vi "AI Driver Initialize.vi"(8 "error in (no error)":errorcluster, 11 "Channel Refs":T3[](array[typedef]) format="%.0x") -> (0 "error out":errorcluster, 3 "Tasks":T1[](array[typedef]))   [LabVIEW 2013]
uses:
  <vilib>/K2Labs/HiLab API/Custom Device API/Controls/Custom Device Item Reference.ctl
  Controls/AI Device Settings.ctl
  Controls/AI Scale.ctl
  <vilib>/K2Labs/HiLab API/Custom Device API/Configuration/Item Properties/Get Item Property/Get Item Property.xnode
  <vilib>/K2Labs/HiLab API/Custom Device API/Custom Device API Library.lvlib
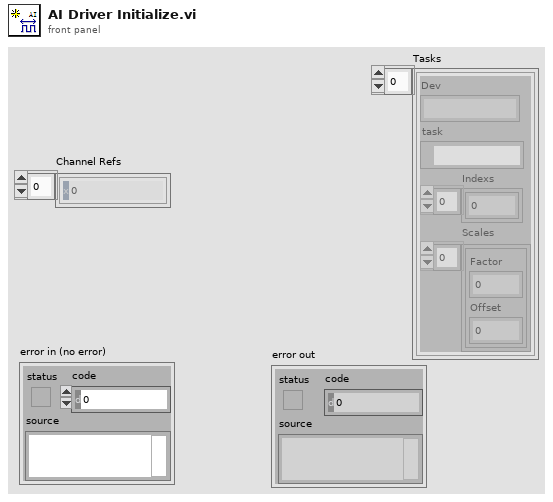
[diagram p1: front panel]
types:
  T1 = typedef "AI Device Settings.ctl" = cluster{"Dev":string, "task":refnum<k21>, "Indexs":i32[], "Scales":T2[]}
  T2 = typedef "AI Scale.ctl" = cluster{"Factor":dbl, "Offset":dbl}
  T3 = typedef "Custom Device API Library.lvlib/Custom Device Item Reference.ctl" = u64
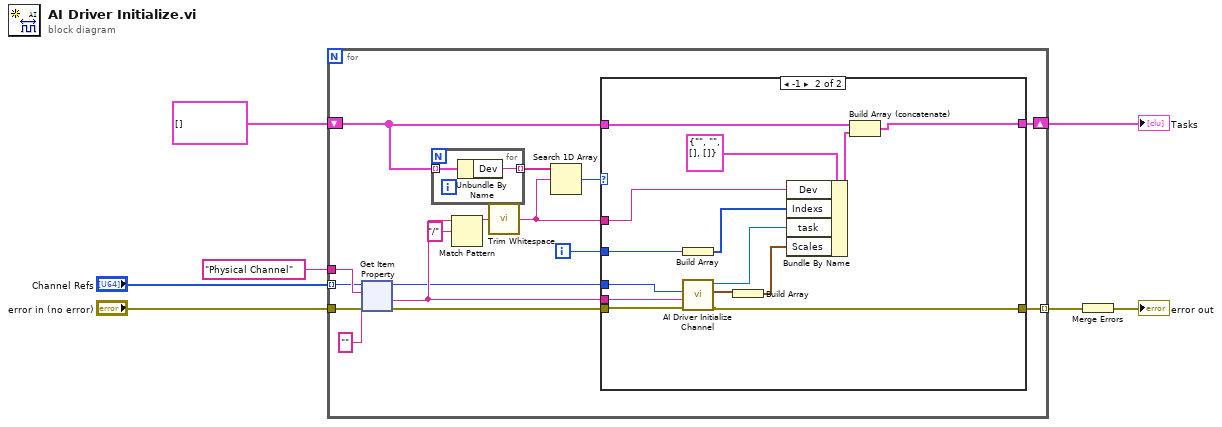
[diagram p0: block diagram]
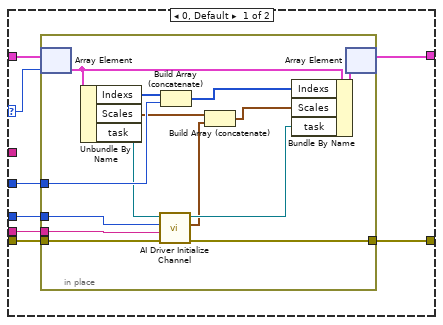
[diagram p2: hidden frame]
diagram:
  n1 = for {
    tunnel: "Physical Channel" ("Property Name") -> [w23]
    tunnel: "Channel Refs" -> [w22] mode=indexing
    shift-right: [w16] -> w1
    shift-left: T1[] [] -> [w17]
    tunnel: [w11] -> w3 mode=indexing
    tunnel: "error in (no error)" -> [w10]
    i -> [w12]
    n2 = xnode "Get Item Property"("Item Ref in"=w22, "Property Name"=w23, "Default Value"="", "error in (no error)"=w10) -> ("Item Ref out"=w9:T3, "Value"=w14:string, "error out"=w13:errorcluster)  [unwired: 1 out]
    n3 = for {
      tunnel: w17 -> [w92] mode=indexing
      tunnel: [w91] -> w20 mode=indexing
      n4 = Unbundle By Name(w92) -> ("Dev"=w91:string)
    }
    n5 = Match Pattern(string=w14, regular expression="/" ("正则表达式")) -> (before substring=w19:string)  [unwired: 1 in, 3 out]
    n6 = call <vilib>:"Trim Whitespace.vi"("string"=w19) -> ("trimmed string"=w15:string)  [unwired: 1 in]
    n7 = Search 1D Array(1D array=w20, element=w15) -> (index of element=w18:i32)  [unwired: 1 in]
    n8 = case shown="-1" w18 {
      selector: w18 -> [w61 _]
      tunnel: w17 -> [w62 w90]
      tunnel: [w56 w89] -> w16
      tunnel: w15 -> [_ w87]
      tunnel: w14 -> [w60 w83]
      tunnel: w13 -> [w59 w82]
      tunnel: w12 -> [w57 w86]
      tunnel: [w58 w81] -> w11
      tunnel: w9 -> [w55 w84]
      frame 0, Default {
        n9 = in-place {
          in-place-border: w60 -> [w68]
          in-place-border: w59 -> [w67]
          in-place-border: [w66] -> w58
          in-place-border: w57 -> [w75]
          in-place-border: w55 -> [w69]
          n10 = in-place-array #1(w62, w61) -> (w74:T1)
          n11 = Unbundle By Name(w74) -> ("Indexs"=w76:i32[], "Scales"=w65:T2[], "task"=w71:refnum<k21>)
          n12 = call "AI Driver Initialize Channel.vi"("错误输入（无错误）"=w67, "Physical Channel"=w68, "Channel Ref"=w69, "Task in"=w71) -> ("错误输出"=w66:errorcluster, "Scale"=w64:T2, "Task out"=w70:refnum<k21>)  [unwired: 5 in]
          n13 = Build Array (concatenate)(w76, w75) -> (w73:i32[])
          n14 = Build Array (concatenate)(w65, w64) -> (w63:T2[])
          n15 = Bundle By Name(cluster=w74, "Indexs"=w73, "Scales"=w63, "task"=w70) -> (w72:T1)
          n16 = in-place-array #1(w72) -> (w56:T1[])  [unwired: 1 out]
        }
      }
      frame -1 {
        n17 = Build Array(w86) -> (w85:i32[])
        n18 = call "AI Driver Initialize Channel.vi"("错误输入（无错误）"=w82, "Physical Channel"=w83, "Channel Ref"=w84) -> ("错误输出"=w81:errorcluster, "Scale"=w78:T2, "Task out"=w80:refnum<k21>)  [unwired: 6 in]
        n19 = Build Array(w78) -> (w77:T2[])
        n20 = Bundle By Name(cluster=T1 {"Dev"="", "task"="", "Indexs"=[], "Scales"=[]}, "Dev"=w87, "Indexs"=w85, "task"=w80, "Scales"=w77) -> (w88:T1)
        n21 = Build Array (concatenate)(w90, w88) -> (w89:T1[])
      }
    }
  }
  "Tasks" <- w1
  n22 = Merge Errors(w3) -> (→"error out":errorcluster)
